vi "DataBase Queue - Dequeue.vi"(8 "error in":errorcluster) -> (0 "error out":errorcluster, 1 "Message Data":variant, 2 "Message":string)   [LabVIEW 2024, in "Data Base.lvlib"]
uses:
  Data Base.lvlib
  Support/General Type Defs/FGV States.ctl
  Support/QMH Messaging/QMH - Dequeue Element.vi
  Support/QMH Messaging/QMH Messaging.lvlib
  Support/General Type Defs/General Type Definitions.lvlib
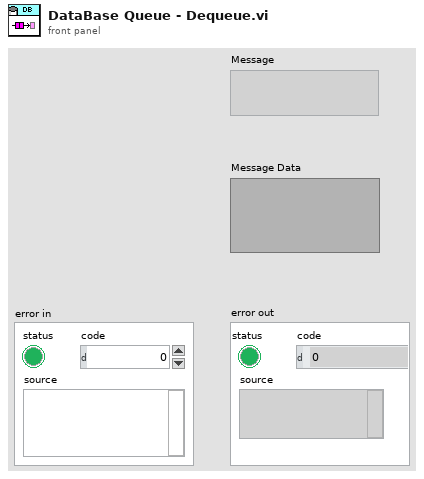
[diagram p1: front panel]
types:
  T1 = typedef "General Type Definitions.lvlib/FGV States.ctl" = enum16{"Create", "Get", "Destroy"}
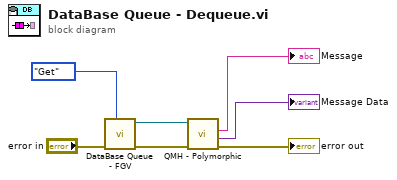
[diagram p0: block diagram]
diagram:
  n1 = call "DataBase Queue - FGV.vi"("FGV States"=FGV_States."Get", "error in"="error in") -> ("error out"=w6:errorcluster, "queue out"=w7:refnum<queue>)  [unwired: 8 in]
  n2 = call-poly "QMH - Polymorphic.vi"("error in (no error)"=w6, "Message Queue"=w7) -> ("error out"=→"error out":errorcluster, "Message Data"=→"Message Data":variant, "Message"=→"Message":string)  [unwired: 6 in, 1 out]
